vi "Print CD Error.vi"(5 "Custom Device? (T)":bool=TRUE, 7 "error in":errorcluster, 10 "Your code's public name":string) -> (0 "error out":errorcluster)   [LabVIEW 2015, in "Engine Simulation Toolkit Engine.lvlib"]
doc: "Prints error information out to the console. Provide your code's public name. For example, if your code is about J1939, put that here so the user knows what this printed error information has to do with.\n\nIf this is not a NI VeriStand custom device, write false to the Custom Device? input. This will change the error output.\n\nIf the 'note' field is empty, it is not printed to the console.\n\nExample output 1:\n******J1939 ERROR******\nSource: blah.vi\nCode: 535\n******J1939 ERROR******\n\nExample output 2:\n******XCP and CCP Master CUSTOM DEVICE ERROR******\nSource: blah.vi\nCode: 535\nUser Note: before write\n******XCP and CCP Master CUSTOM DEVICE ERROR******"
uses:
  Engine Simulation Toolkit Engine.lvlib
  <vilib>/Utility/error.llb/DialogType.ctl
  <vilib>/NI Veristand/Custom Device Tools/Custom Device Utility Library/RT Debug String Color Spec.ctl
  <vilib>/NI Veristand/Custom Device Tools/Custom Device Utility Library/Custom Device Utility Library.lvlib
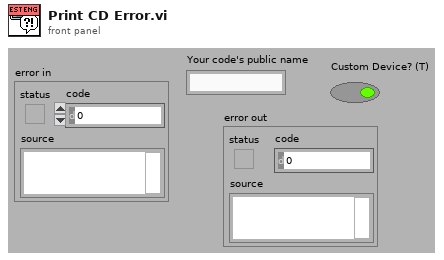
[diagram p1: front panel]
types:
  T1 = typedef "Custom Device Utility Library.lvlib/RT Debug String Color Spec.ctl" = u16
  T2 = typedef "DialogType.ctl" = u16
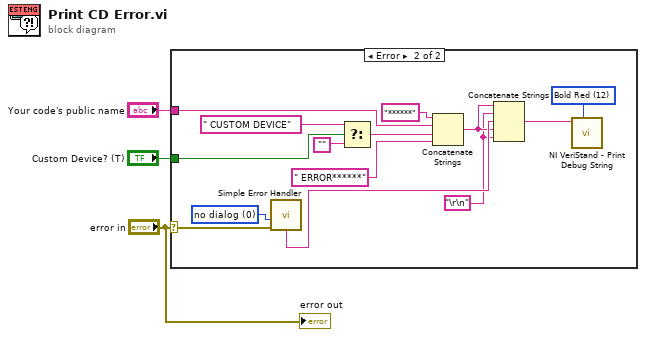
[diagram p0: block diagram]
diagram:
  n1 = case shown="Error" "error in" {
    selector: "error in" -> [_ w11]
    tunnel: "Custom Device? (T)" -> [_ w12]
    tunnel: "Your code's public name" -> [_ w6]
    frame No Error {
    }
    frame Error {
      w4 = T1 12 items=["Plain White"=7, "Bold White"=15, "Bold Blue"=9, "Bold Green"=10, "Bold Red"=12] ("Attribute")
      w10 = T2 0 items=["no dialog", "OK message", "continue or stop message", "OK message + warnings", "continue/stop + warnings"] ("type of dialog (OK msg:1)")
      w7 = "\r\n"
      n2 = call <vilib>:"Simple Error Handler.vi"("type of dialog (OK msg:1)"=w10, "error in (no error)"=w11) -> ("message"=w9:string)  [unwired: 3 in, 4 out]
      n3 = Select(t=" CUSTOM DEVICE" ("String"), s=w12, f="") -> (s? t:f=w13:string)
      n4 = Concatenate Strings("******" ("String"), w6, w13, " ERROR******" ("String")) -> (w8:string)
      n5 = Concatenate Strings(w8, w7, w9, w8, w7) -> (w5:string)
      n6 = call <vilib>:"NI VeriStand - Print Debug String.vi"("Attribute"=w4, "Message"=w5) -> ()  [unwired: 9 in, 1 out]
    }
  }
  "error out" <- "error in"
